vi "Execute Command (2D string results).vi"(8 "error in (no error)":errorcluster, 9 "Parameters":variant, 10 "SQL":string, 11 "PQ Connection in":refnum<class "PQ Connection.lvclass">) -> (0 "error out":errorcluster, 1 "Result":string[][](array[string]), 2 "Number of Rows":i32, 3 "PQ Connection out":refnum<class "PQ Connection.lvclass">)   [LabVIEW 2015, in "PQ Connection.lvclass"]
doc: "Execute one or more SQL commands. Optionally, one can provide parameters to be bound to $n tokens in the SQL command (eg. \"SELECT * FROM mytable WHERE x = $1\"). If parameters are provided than only one SQL command can be executed. The parameters can be a cluster or an array, or can be a single value if only one parameter is needed.\n\nResults (of the first command to return results) are provided as a 2D array of strings."
uses:
  PQ Connection.lvclass
  Result/PQ Result.lvclass/PQ Result.ctl
  Single Command with parameters.vi
  Execute (Return first result with rows).vi
  Result/PQ Result.lvclass
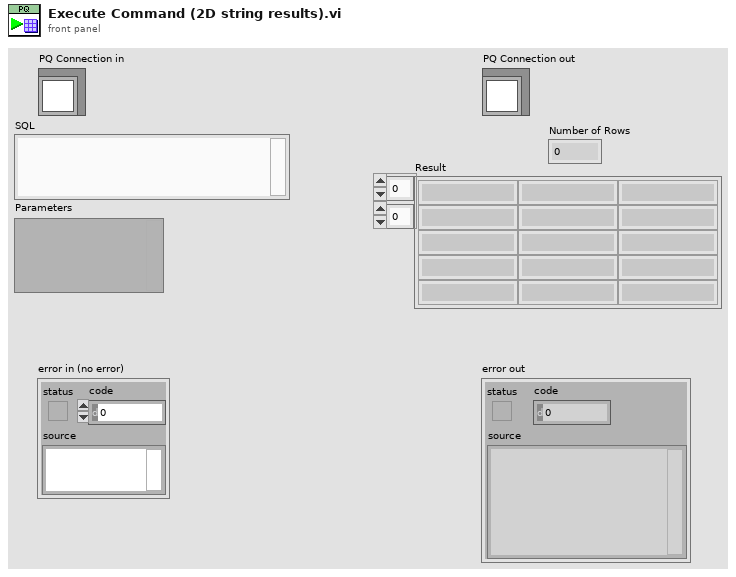
[diagram p1: front panel]
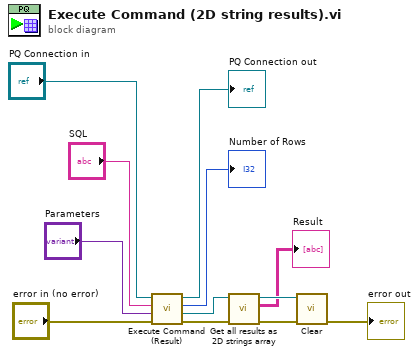
[diagram p0: block diagram]
diagram:
  n1 = call "Execute Command (Result).vi"("error in (no error)"="error in (no error)", "Parameter(s)"="Parameters", "SQL"="SQL", "PQ Connection in"="PQ Connection in") -> ("error out"=w6:errorcluster, "First Result with Rows returned"=w5:refnum<class "PQ Result.lvclass">, "Number of Rows"=→"Number of Rows":i32, "PQ Connection out"=→"PQ Connection out":refnum<class "PQ Connection.lvclass">)  [unwired: 4 in]
  n2 = call "Get all results as 2D strings array.vi"("error in (no error)"=w6, "PQ Result in"=w5) -> ("error out"=w3:errorcluster, "Strings"=→"Result":string[][], "PQ Result out"=w4:refnum<class "PQ Result.lvclass">)  [unwired: 7 in]
  n3 = call "Clear.vi"("error in (no error)"=w3, "PQ Result  in"=w4) -> ("error out"=→"error out":errorcluster)  [unwired: 9 in]
